vi "Do.vi"(8 "error in (no error)":errorcluster, 9 "CommandQueueIn":refnum<queue>, 10 "DataNotifierIn":refnum<notifier>, 11 "CommandCopy in":refnum<class "Initialize.lvclass">) -> (0 "error out":errorcluster, 1 "ExitFlag":bool, 2 "DataNotifierOut":refnum<notifier>, 3 "CommandCopy out":refnum<class "Initialize.lvclass">)   [LabVIEW 2013, in "Initialize.lvclass"]
uses:
  Initialize.lvclass
  SystemData.lvclass/SystemData.lvclass
  RootCommand.lvclass/RootCommand.lvclass
  GenSin.lvclass/GenSin.lvclass
  GenSquare.lvclass/GenSquare.lvclass
  GenTriangle.lvclass/GenTriangle.lvclass
  SystemData.lvclass/SystemData.lvclass/SystemData.ctl
  Generator.lvclass/Generator.lvclass
panel:
  # "notifier包裝SystemData物件的參考"
  # "命令物件序列參考"
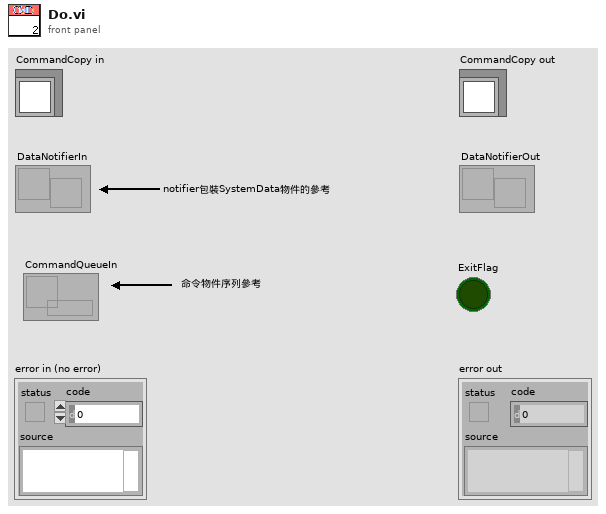
[diagram p1: front panel]
types:
  T1 = typedef "SystemData.lvclass/SystemDataTypeDefine.ctl" = cluster{"ThisVIParameter":cluster{"ThisVIPath":path, "ThisVIReference":refnum<vi>, "AllControlReference":refnum<vi>[]}, "GeneratorParameter":cluster{"Frequency":dbl, "Amplitude":dbl}, "WaveformBuffer":waveform(dbl), "SourceSelect":u16, "GeneratorClassArray":refnum<class "Generator.lvclass">[]}
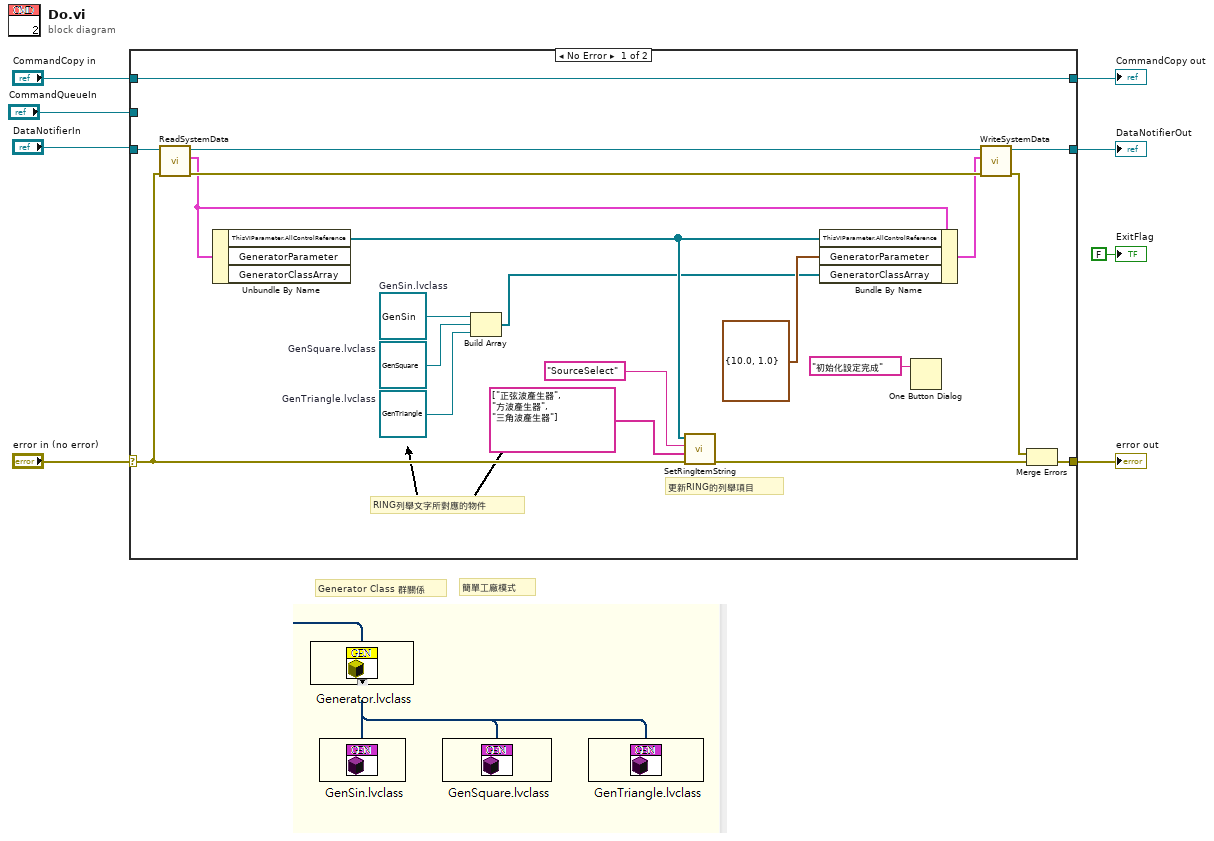
[diagram p0: block diagram]
diagram:
  # "簡單工廠模式"
  # "Generator Class 群關係"
  n1 = case shown="No Error" "error in (no error)" {
    selector: "error in (no error)" -> [w21 w31]
    tunnel: [w20 w31] -> w4
    tunnel: [w28 w30] -> w3
    tunnel: "CommandCopy in" -> [w28 w30]
    tunnel: "DataNotifierIn" -> [w27 w29]
    tunnel: [w22 w29] -> w2
    tunnel: "CommandQueueIn" -> [_ _]
    frame No Error {
      w10 = refnum<class "GenTriangle.lvclass"> refnum  # GenTriangle.lvclass
      w12 = refnum<class "GenSquare.lvclass"> refnum  # GenSquare.lvclass
      w11 = refnum<class "GenSin.lvclass"> refnum  # GenSin.lvclass
      # "更新RING的列舉項目"
      # "RING列舉文字所對應的物件"
      n2 = call "ReadSystemData.vi"("error in (no error)"=w21, "DataNotifierIn"=w27) -> ("error out"=w25:errorcluster, "SystemData"=w24:T1, "DataNotifierIn"=w26:refnum<notifier>)  [unwired: 7 in]
      n3 = Unbundle By Name(w24) -> ("ThisVIParameter.AllControlReference"=w16:refnum<vi>[])  [unwired: 2 out]
      n4 = Build Array(w11, w12, w10) -> (w9:refnum<class "Generator.lvclass">[])
      n5 = call "SetRingItemString.vi"("error in (no error)"=w21, "Strings []"=string[] ["正弦波產生器", "方波產生器", "三角波產生器"], "TargetCtlLabel.Text"="SourceSelect", "AllControlReference"=w16) -> ("error out"=w18:errorcluster)  [unwired: 7 in]
      n6 = Bundle By Name(cluster=w24, "ThisVIParameter.AllControlReference"=w16, "GeneratorParameter"=cluster{"Frequency":dbl, "Amplitude":dbl} {"Frequency"=10.0, "Amplitude"=1.0}, "GeneratorClassArray"=w9) -> (w23:T1)
      n7 = One Button Dialog(message="初始化設定完成") -> ()  [unwired: 1 in, 1 out]
      n8 = call "WriteSystemData.vi"("error in (no error)"=w25, "SystemData"=w23, "DataNotifierIn"=w26) -> ("error out"=w19:errorcluster, "DataNotifierOut"=w22:refnum<notifier>)  [unwired: 7 in]
      n9 = Merge Errors(w19, w18) -> (w20:errorcluster)
    }
    frame Error {
    }
  }
  "error out" <- w4
  "CommandCopy out" <- w3
  "DataNotifierOut" <- w2
  "ExitFlag" <- FALSE ("ExitFlag")
